vi "Set Intensity Graph Value.vi"(9 "Data Updated":dbl[][](array[numeric]) format="%#_f", 11 "Ref In":refnum<vi>) -> ()   [LabVIEW 2024]
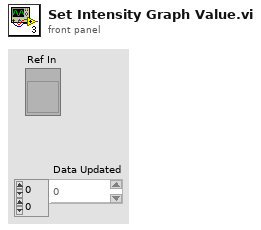
[diagram p1: front panel]
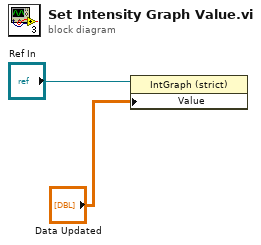
[diagram p0: block diagram]
diagram:
  n1 = property class="IntGraph (strict)"(reference="Ref In", "Value"="Data Updated") -> ()  [unwired: 1 in, 2 out]
